vi "_loadCamera.vi"(4 "error in (no error)":errorcluster, 6 "camera select":T1, 7 "_cameraBase.lvclass":refnum<class "_cameraBase.lvclass">) -> (0 "error out":errorcluster, 3 "_cameraBase.lvclass":refnum<class "_cameraBase.lvclass">)   [LabVIEW 2019, in "_cameraBase.lvclass"]
uses:
  _cameraBase.lvclass
  camType.ctl
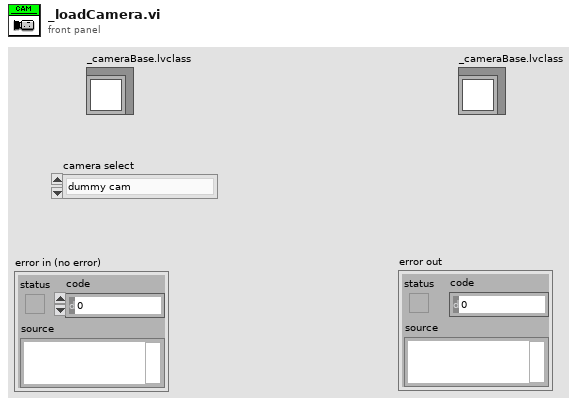
[diagram p1: front panel]
types:
  T1 = typedef "camType.ctl" = enum16{"dummy cam", "StresingDualCam"}
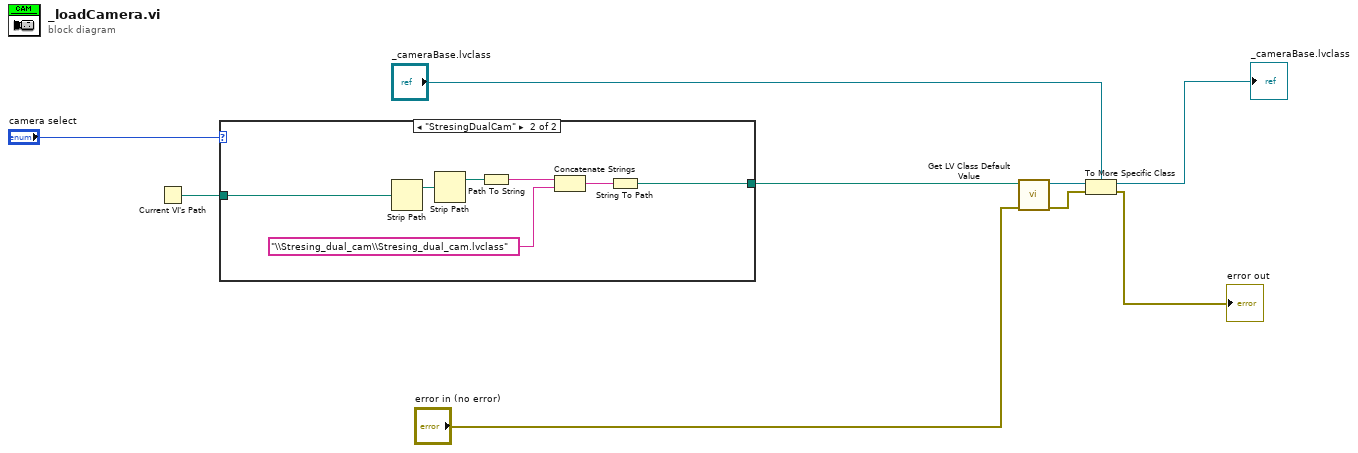
[diagram p0: block diagram]
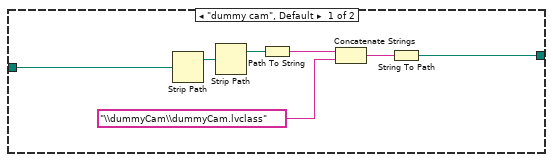
[diagram p2: hidden frame]
diagram:
  n1 = Current VI's Path() -> (path=w2:path)
  n2 = case shown="\"StresingDualCam\"" "camera select" {
    tunnel: [w11 w17] -> w3
    tunnel: w2 -> [w10 w18]
    frame "dummy cam", Default {
      n3 = Strip Path(path=w10) -> (stripped path=w16:path)  [unwired: 1 out]
      n4 = Strip Path(path=w16) -> (stripped path=w15:path)  [unwired: 1 out]
      n5 = Path To String(path=w15) -> (string=w14:string)
      n6 = Concatenate Strings(w14, "\\dummyCam\\dummyCam.lvclass") -> (w12:string)
      n7 = String To Path(string=w12) -> (path=w11:path)
    }
    frame "StresingDualCam" {
      n8 = Strip Path(path=w18) -> (stripped path=w23:path)  [unwired: 1 out]
      n9 = Strip Path(path=w23) -> (stripped path=w22:path)  [unwired: 1 out]
      n10 = Path To String(path=w22) -> (string=w21:string)
      n11 = Concatenate Strings(w21, "\\Stresing_dual_cam\\Stresing_dual_cam.lvclass") -> (w19:string)
      n12 = String To Path(string=w19) -> (path=w17:path)
    }
  }
  n13 = call <vilib>:"Get LV Class Default Value.vi"("error in (no error)"="error in (no error)", "class path"=w3) -> ("error out"=w7:errorcluster, "object"=w4:refnum<class>)  [unwired: 8 in]
  n14 = To More Specific Class(target class="_cameraBase.lvclass", reference=w4, error in=w7) -> (specific class reference=→"_cameraBase.lvclass":refnum<class "_cameraBase.lvclass">, error out=→"error out":errorcluster)
